vi "Controller to Boiler.vi"(7 "Notifier":refnum<notifier>, 8 "error in":errorcluster, 9 "Message Data":variant, 10 "Message":string="Run Interlock", 11 "Boiler Queue in":refnum<queue>) -> (0 "error out":errorcluster, 2 "notification":variant, 3 "Queue out":refnum<queue>)   [LabVIEW 2015]
doc: "Send a command to the boiler and wait for it to be executed."
uses:
  Message Queue/Message Cluster.ctl
  Message Queue/Message Queue.lvlib
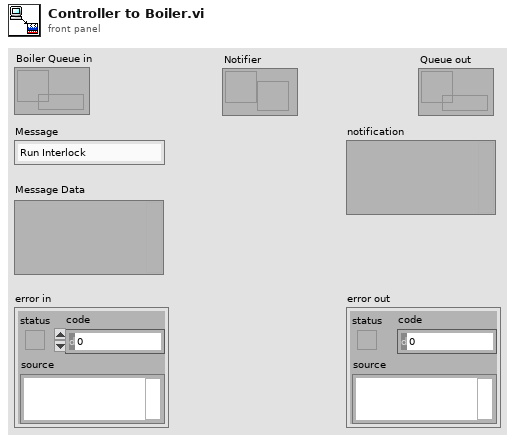
[diagram p1: front panel]
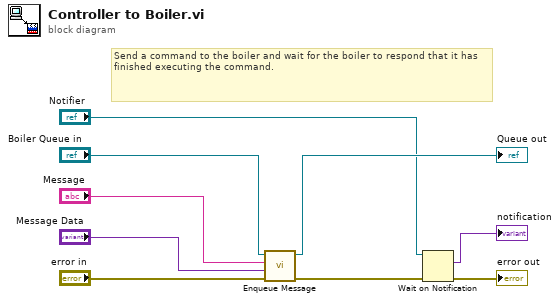
[diagram p0: block diagram]
diagram:
  # "Send a command to the boiler and wait for the boiler to respond that it has finished executing the command."
  n1 = call "Enqueue Message.vi"("error in (no error)"="error in", "Message Data"="Message Data", "Message"="Message", "Message Queue"="Boiler Queue in") -> ("error out"=w2:errorcluster, "dup Message Queue"=→"Queue out":refnum<queue>)  [unwired: 6 in]
  n2 = Wait on Notification(notifier="Notifier", error in (no error)=w2) -> (notification=→"notification":variant, error out=→"error out":errorcluster)  [unwired: 2 in, 2 out]
